vi "benchmark-QMH.vi"(11 "iterations":i32=100000) -> (2 "duration (s)":dbl, 3 "data":dbl[][](array[numeric]))   [LabVIEW 2020]
uses:
  <vilib>/Analysis/baseanly.llb/Mean (DBL).vi
  <vilib>/Analysis/NI_AALBase.lvlib
panel:
  out "loop delay":dbl[][](graph)
  out "max value 2":dbl format="%#_6f"
  out "min value 2":dbl format="%#_6f"
  out "mean 2":dbl format="%#_6f"
  out "valid":bool
  out "error out":errorcluster
  out "mean":dbl format="%#_6f"
  out "min value":dbl format="%#_6f"
  out "max value":dbl format="%#_6f"
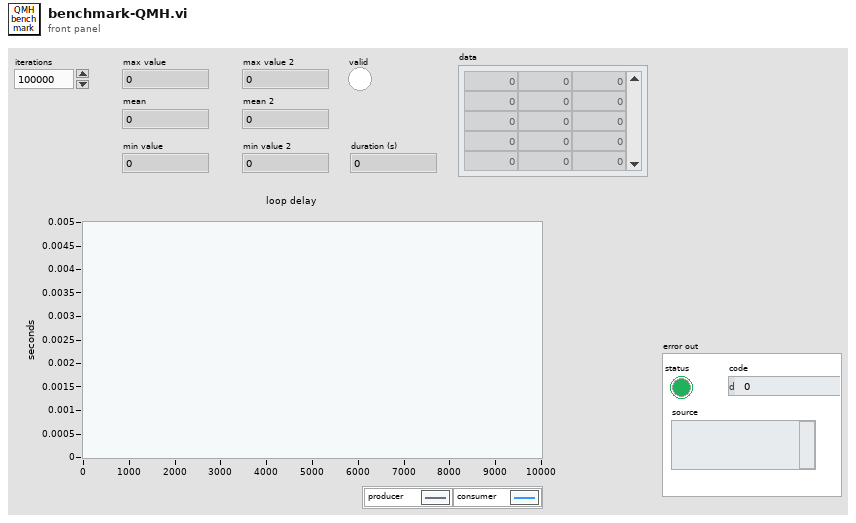
[diagram p1: front panel]
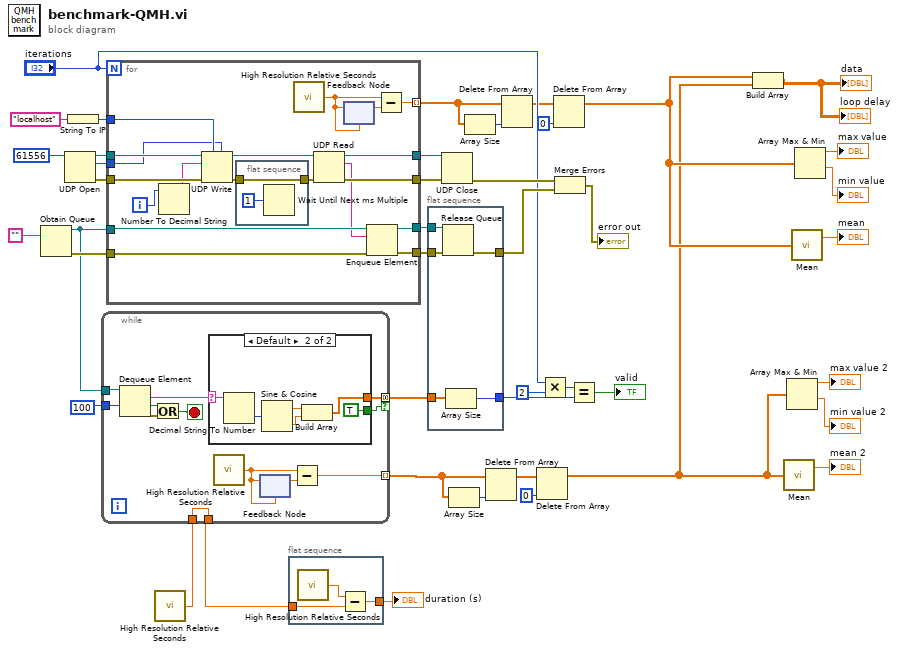
[diagram p0: block diagram]
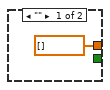
[diagram p2: hidden frame]
diagram:
  n1 = Obtain Queue(element data type="") -> (queue out=w5:refnum<queue>, error out=w29:errorcluster)  [unwired: 4 in, 1 out]
  n2 = UDP Open(11:u16 61556 ("port")) -> (port=w36:refnum<k16>, 0:w35:errorcluster, 2:w31:u16)  [unwired: 4 in]
  n3 = String To IP(1:"localhost" ("service name")) -> (0:w32:u32)
  n4 = for {
    N: "iterations" -> [_]
    tunnel: [w61] -> w6 mode=indexing
    tunnel: [w58] -> w38
    tunnel: [w57] -> w37
    tunnel: w36 -> [w56]
    tunnel: w35 -> [w55]
    tunnel: w32 -> [w52]
    tunnel: w31 -> [w51]
    tunnel: w5 -> [w50]
    tunnel: [w48] -> w28
    tunnel: w29 -> [w47]
    tunnel: [w46] -> w27
    i -> [w54]
    n5 = Number To Decimal String(number=w54) -> (decimal integer string=w53:string)  [unwired: 1 in]
    n6 = UDP Write(address=w52, port or service name=w51, connection ID=w56, data in=w53, 8:w55) -> (error out=w45:errorcluster, 3:w59:refnum<k16>)  [unwired: 1 in]
    n7 = flat-sequence {
      tunnel: w45 -> [w64]
      tunnel: [w64] -> w44
      frame #0 {
        n8 = Wait Until Next ms Multiple(millisecond multiple=u32 1) -> ()  [unwired: 1 out]
      }
    }
    n9 = call <vilib>:"High Resolution Relative Seconds.vi"() -> ("relative seconds"=w60:dbl)
    n10 = UDP Read(connection ID=w59, 8:w44) -> (data out=w49:string, error out=w58:errorcluster, 3:w57:refnum<k16>)  [unwired: 2 in, 2 out]
    n11 = feedback #1(w60) -> (w62:dbl)
    n12 = feedback-in #1(w60) -> ()
    n13 = Enqueue Element(queue=w50, element=w49, error in (no error)=w47) -> (queue out=w48:refnum<queue>, error out=w46:errorcluster)  [unwired: 1 in, 1 out]
    n14 = Subtract(x=w60, y=w62) -> (x-y=w61:dbl)
  }
  n15 = call <vilib>:"High Resolution Relative Seconds.vi"() -> ("relative seconds"=w3:dbl)
  n16 = while {
    tunnel: w5 -> [w76]
    tunnel: [w74] -> w23 mode=concatenating if=w73
    tunnel: 100 ("timeout in ms (-1)") -> [w72]
    tunnel: [w66] -> w17 mode=indexing
    tunnel: w3 -> [w65]
    tunnel: [w65] -> w2
    stop <- w69 stop-if-true
    n17 = Dequeue Element(queue=w76, timeout in ms (-1)=w72) -> (element=w75:string, timed out?=w71:bool, error out=w70:errorcluster)  [unwired: 1 in, 1 out]
    n18 = Or(x=w71, y=w70) -> (x .or. y?=w69:bool)
    n19 = case shown="Default" w75 {
      selector: w75 -> [_ w83]
      tunnel: [dbl[] [] w80] -> w74
      tunnel: [_ TRUE] -> w73
      frame "" {
      }
      frame Default {
        n20 = Decimal String To Number(string=w83) -> (number=w78:i32)  [unwired: 2 in, 1 out]
        n21 = Sine & Cosine(0:w78) -> (1:w82:dbl, 2:w81:dbl)
        n22 = Build Array(w82, w81) -> (w80:dbl[])
      }
    }
    n23 = call <vilib>:"High Resolution Relative Seconds.vi"() -> ("relative seconds"=w68:dbl)
    n24 = feedback #2(w68) -> (w67:dbl)
    n25 = feedback-in #2(w68) -> ()
    n26 = Subtract(x=w68, y=w67) -> (x-y=w66:dbl)
  }
  n27 = flat-sequence {
    tunnel: w2 -> [w85]
    tunnel: [w84] -> w4
    frame #0 {
      n28 = call <vilib>:"High Resolution Relative Seconds.vi"() -> ("relative seconds"=w86:dbl)
      n29 = Subtract(x=w86, y=w85) -> (x-y=w84:dbl)
    }
  }
  n30 = flat-sequence {
    tunnel: w28 -> [w91]
    tunnel: w27 -> [w90]
    tunnel: [w89] -> w25
    tunnel: w23 -> [w88]
    tunnel: [w87] -> w20
    frame #0 {
      n31 = Release Queue(queue=w91, error in (no error)=w90) -> (error out=w89:errorcluster)  [unwired: 1 in, 2 out]
      n32 = Array Size(array=w88) -> (size(s)=w87:i32)
    }
  }
  n33 = UDP Close(connection ID=w37, 8:w38) -> (error out=w26:errorcluster)  [unwired: 1 out]
  n34 = Array Size(array=w17) -> (size(s)=w12:i32)
  n35 = Array Size(array=w6) -> (size(s)=w8:i32)
  n36 = Delete From Array(array=w17, index=w12) -> (array with subset deleted=w11:dbl[])  [unwired: 1 in, 1 out]
  n37 = Delete From Array(array=w6, index=w8) -> (array with subset deleted=w7:dbl[])  [unwired: 1 in, 1 out]
  n38 = Delete From Array(array=w11, index=0) -> (array with subset deleted=w9:dbl[])  [unwired: 1 in, 1 out]
  n39 = Multiply(x="iterations", y=2) -> (x*y=w21:i32)
  n40 = Delete From Array(array=w7, index=0) -> (array with subset deleted=w39:dbl[])  [unwired: 1 in, 1 out]
  n41 = Merge Errors(w26, w25) -> (→"error out":errorcluster)
  n42 = Equal?(x=w21, y=w20) -> (x = y?=→"valid":bool)
  n43 = Build Array(w39, w9) -> (→"data" →"loop delay":dbl[][])
  n44 = call-poly <vilib>:"Mean.vi"("X"=w9) -> ("mean"=→"mean 2":dbl)  [unwired: 1 out]
  n45 = Array Max & Min(array=w9) -> (max value=→"max value 2":dbl, min value=→"min value 2":dbl)  [unwired: 2 out]
  n46 = call-poly <vilib>:"Mean.vi"("X"=w39) -> ("mean"=→"mean":dbl)  [unwired: 1 out]
  n47 = Array Max & Min(array=w39) -> (max value=→"max value":dbl, min value=→"min value":dbl)  [unwired: 2 out]
  "duration (s)" <- w4
